vi "Measure Zero Span.vi"(8 "error in (no error)":errorcluster, 10 "Center Frequency (Hz)":dbl=1000000000.0 format="%_9p", 11 "Instrument.lvclass in":refnum<class "Instrument.lvclass">) -> (0 "error out":errorcluster, 1 "Marker Position (Delta Hz)":dbl format="%#_6p", 2 "Marker Amplitude (dBm)":dbl format="%#_6f", 3 "Instrument.lvclass out":refnum<class "Instrument.lvclass">)   [LabVIEW 2014, in "Instrument.lvclass"]
uses:
  Instrument.lvclass
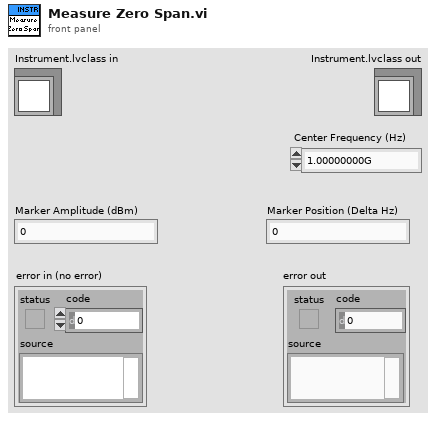
[diagram p1: front panel]
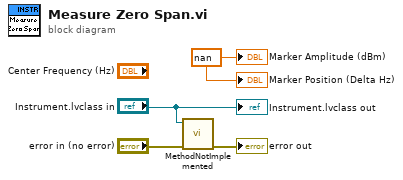
[diagram p0: block diagram]
diagram:
  w2 = nan ("Marker Amplitude (dBm)")
  n1 = call "MethodNotImplemented.vi"("error in (no error)"="error in (no error)", "LabVIEW Object In"="Instrument.lvclass in") -> ("error out"=→"error out":errorcluster)  [unwired: 9 in]
  "Marker Position (Delta Hz)" <- w2
  "Marker Amplitude (dBm)" <- w2
  "Instrument.lvclass out" <- "Instrument.lvclass in"
